vi "Select Channel.vi"(1 "Ch In":u8) -> (0 "Chip Select":T1=enum."None")   [LabVIEW 2018]
uses:
  Type Defs/Chip Select.ctl
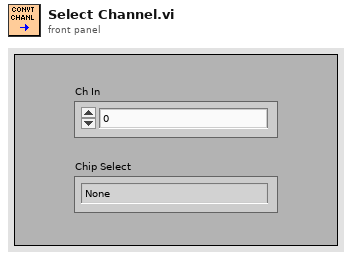
[diagram p1: front panel]
types:
  T1 = typedef "Chip Select.ctl" = enum16{"Axial Field", "None", "dsPIC Corona"}
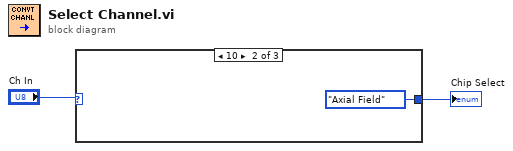
[diagram p0: block diagram]
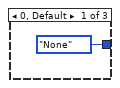
[diagram p2: hidden frame]
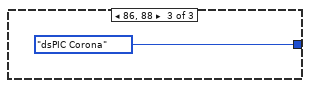
[diagram p3: hidden frame]
diagram:
  n1 = case shown="10" "Ch In" {
    tunnel: [Chip_Select."None" ("Chip Select") Chip_Select."Axial Field" ("Chip Select") Chip_Select."dsPIC Corona" ("Chip Select")] -> w1
    frame 0, Default {
    }
    frame 10 {
    }
    frame 86, 88 {
    }
  }
  "Chip Select" <- w1
